vi "DUAL GAUGE-Reset.vi"(8 "Fehler (Eingang)":errorcluster, 11 "Referenz in":refnum<visa-resource-name>) -> (0 "Cluster (Ausgang)":errorcluster, 1 "Errortext":string[](array[string]), 3 "Referenz out":refnum<visa-resource-name>)   [LabVIEW 2010, in "Dual Gauge.lvlib"]
uses:
  Dual Gauge.lvlib
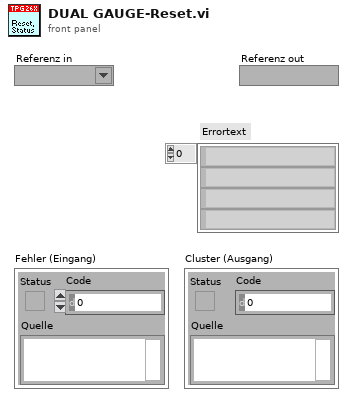
[diagram p1: front panel]
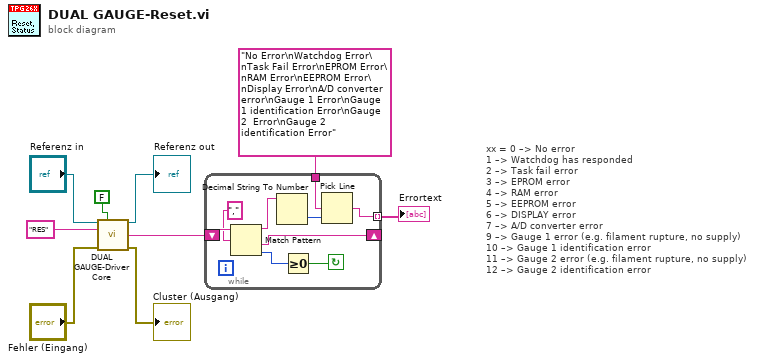
[diagram p0: block diagram]
diagram:
  # "xx = 0 –> No error\n1 –> Watchdog has responded\n2 –> Task fail error\n3 –> EPROM error\n4 –> RAM error\n5 –> EEPROM error\n6 –> DISPLAY error\n7 –> A/D converter error\n9 –> Gauge 1 error (e.g. filament rupture, no supply)\n10 –> Gauge 1 identification error\n11 –> Gauge 2 error (e.g. filament rupture, no supply)\n12 –> Gauge 2 identification error"
  n1 = call "DUAL GAUGE-Driver Core.vi"("Referenz in"="Referenz in", "Write/Read"=FALSE, "Command"="RES", "Fehler (Eingang)"="Fehler (Eingang)") -> ("Referenz out"=→"Referenz out":refnum<visa-resource-name>, "String Out"=w7:string, "Cluster (Ausgang)"=→"Cluster (Ausgang)":errorcluster)  [unwired: 9 in]
  n2 = while {
    tunnel: [w10] -> w9 mode=indexing
    shift-left: w7 -> [w18]
    shift-right: [w11] -> _
    tunnel: "No Error\nWatchdog Error\nTask Fail Error\nEPROM Error\nRAM Error\nEEPROM Error\nDisplay Error\nA/D converter error\nGauge 1 Error\nGauge 1 identification Error\nGauge 2  Error\nGauge 2 identification Error" -> [w17]
    stop <- w15 continue-if-true
    n3 = Match Pattern(string=w18, regular expression=",") -> (before substring=w12:string, after substring=w11:string, offset past match=w14:i32)  [unwired: 1 in, 1 out]
    n4 = Decimal String To Number(string=w12) -> (number=w13:i32)  [unwired: 2 in, 1 out]
    n5 = Greater Or Equal To 0?(x=w14) -> (x >= 0?=w15:bool)
    n6 = Pick Line(multi-line string=w17, line index=w13) -> (output string=w10:string)  [unwired: 1 in]
  }
  "Errortext" <- w9
